vi "Status Code.vi"(8 "error in (no error)":errorcluster, 11 "Status Code":i16) -> (0 "error out":errorcluster, 2 "Status Cluster":T1)   [LabVIEW 2016]
uses:
  sniper current tests/Status  Cluster.ctl
panel:
  in  "Mask Unused?":bool=TRUE
  out "Unused status are 0s":i16 format="0b%16b"
  in  "Unused status are 1s":i16=5120 format="0b%16b"
  out "Status Code 2":i16 format="0b%16b"
  out "size(s) 2":i32
  out "size(s)":i32
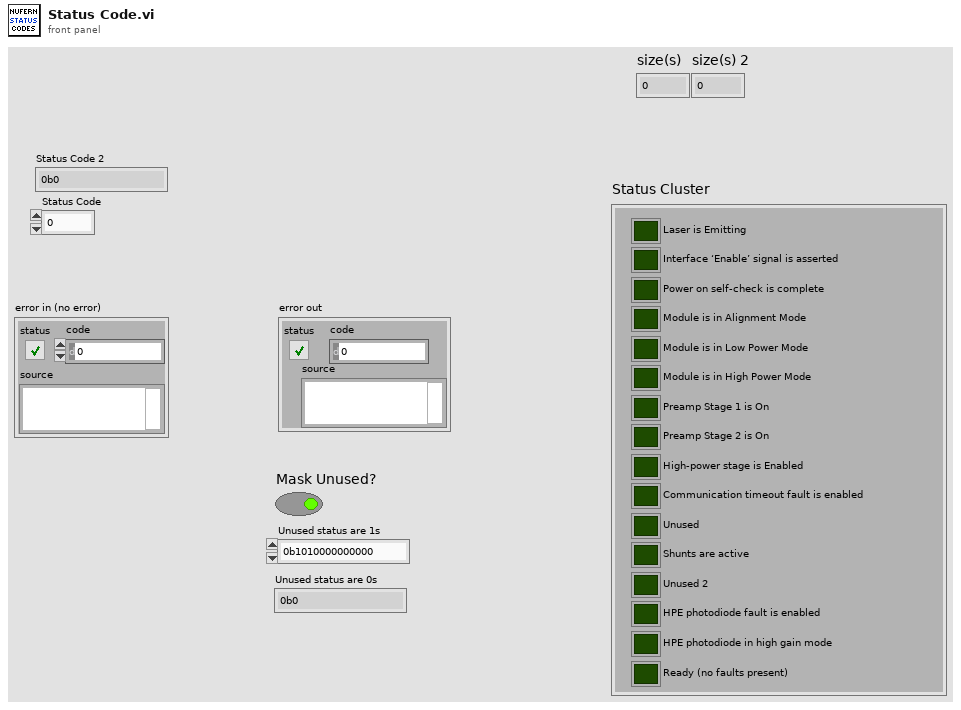
[diagram p1: front panel]
types:
  T1 = typedef "Status  Cluster.ctl" = cluster{"Laser is Emitting":bool, "Interface ‘Enable’ signal is asserted":bool, "Power on self-check is complete":bool, "Module is in Alignment Mode":bool, "Module is in Low Power Mode":bool, "Module is in High Power Mode":bool, "Preamp Stage 1 is On":bool, "Preamp Stage 2 is On":bool, "High-power stage is Enabled":bool, "Communication timeout fault is enabled":bool, "Unused":bool, "Shunts are active":bool, "Unused 2":bool, "HPE photodiode fault is enabled":bool, "HPE photodiode in high gain mode":bool, "Ready (no faults present)":bool}
  T2 = cluster{"[0]":bool, "[1]":bool, "[2]":bool, "[3]":bool, "[4]":bool, "[5]":bool, "[6]":bool, "[7]":bool, "[8]":bool, "[9]":bool, "[10]":bool, "[11]":bool, "[12]":bool, "[13]":bool, "[14]":bool, "[15]":bool}
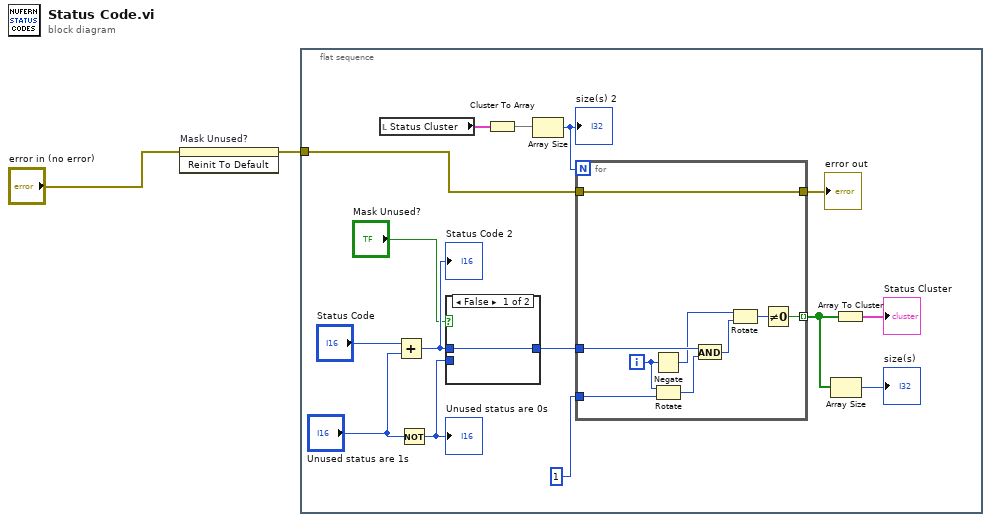
[diagram p0: block diagram]
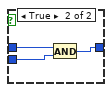
[diagram p2: hidden frame]
diagram:
  n1 = invoke on="Mask Unused?" class="Bool (strict)" method="Reinit To Default"(error in="error in (no error)") -> (error out=w1:errorcluster)  [unwired: 2 in, 2 out]
  n2 = flat-sequence {
    tunnel: w1 -> [w3]
    frame #0 {
      n3 = local read "Status Cluster"() -> (w17:T1)
      n4 = Add(x="Status Code", y="Unused status are 1s") -> (x+y=w6:i16)
      "Status Code 2" <- w6
      n5 = Not(x="Unused status are 1s") -> (.not. x?=w7:i16)
      "Unused status are 0s" <- w7
      n6 = case shown="False" "Mask Unused?" {
        tunnel: [w18 w21] -> w8
        tunnel: w7 -> [_ w20]
        tunnel: w6 -> [w18 w19]
        frame False {
        }
        frame True {
          n7 = And(x=w19, y=w20) -> (x .and. y?=w21:i16)
        }
      }
      n8 = Cluster To Array(cluster=w17) -> (array=w13:bool[])
      n9 = Array Size(array=w13) -> (size(s)=w12:i32)
      "size(s) 2" <- w12
      n10 = for {
        N: w12 -> [_]
        tunnel: w3 -> [w30]
        tunnel: [w30] -> w16
        tunnel: w8 -> [w29]
        tunnel: 1 -> [w28]
        tunnel: [w22] -> w9 mode=indexing
        i -> [w25]
        n11 = Negate(x=w25) -> (-x=w24:i32)
        n12 = Rotate(1:w28, 2:w25) -> (0:w27:i32)
        n13 = And(x=w29, y=w27) -> (x .and. y?=w26:i32)
        n14 = Rotate(1:w26, 2:w24) -> (0:w23:i32)
        n15 = Not Equal To 0?(x=w23) -> (x != 0?=w22:bool)
      }
      "error out" <- w16
      n16 = Array Size(array=w9) -> (size(s)=→"size(s)":i32)
      n17 = Array To Cluster(array=w9) -> (cluster=→"Status Cluster":T2)
    }
  }
